vi "GetImage.vi"(0 "XRef":T5, 1 "State In":T3) -> (14 "Image":T2, 15 "Fatal Error Out":T1)   [LabVIEW 2015, in "LVJSON.lvlib" / "Set Object Parameters.xnode"]
uses:
  Set Object Parameters.xnode
  <vilib>/XNodeSupport/XNodeXNodeRef.ctl
  State.ctl
  Get Object Parameters/Parameter.ctl
  <vilib>/XNodeSupport/XNodeImage.ctl
  <vilib>/XNodeSupport/XNodeErrorCluster.ctl
  Shared/Shared.lvlib
  <vilib>/XNodeSupport/NI_XNodeSupport.lvlib
panel:
  in  "picture":picture
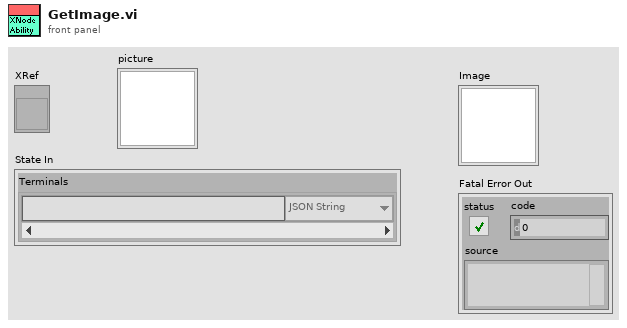
[diagram p1: front panel]
types:
  T1 = typedef "NI_XNodeSupport.lvlib/XNodeErrorCluster.ctl" = errorcluster
  T2 = typedef "NI_XNodeSupport.lvlib/XNodeImage.ctl" = picture
  T3 = typedef "LVJSON.lvlib/Set Object Parameters.xnode/State.ctl" = cluster{"Terminals":T4[]}
  T4 = typedef "LVJSON.lvlib/Shared.lvlib/Parameter.ctl" = cluster{"Parameter Name":string, "JSON Type":enum16{"JSON String", "JSON Numeric", "JSON Boolean", "JSON", "JSON Object", "JSON Array", "String Value", "Numeric Value", "Boolean Value"}}
  T5 = typedef "NI_XNodeSupport.lvlib/XNodeXNodeRef.ctl" = refnum<vi>
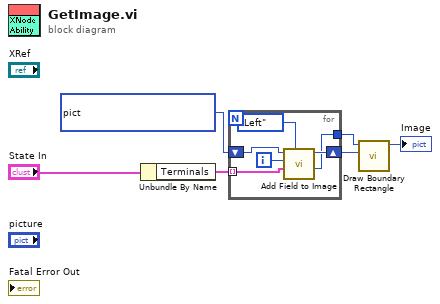
[diagram p0: block diagram]
diagram:
  n1 = Unbundle By Name("State In") -> ("Terminals"=w3:T4[])
  n2 = for {
    shift-right: [w12] -> w5
    shift-left: picture bytes[15070] ("new picture") -> [w11]
    tunnel: w3 -> [w9] mode=indexing
    tunnel: [w8] -> w4
    i -> [w10]
    n3 = call "Add Field to Image.vi"("Justification"=enum16{"Left", "Center", "Right"}."Left", "Terminal Info"=w9, "location"=w10, "picture"=w11) -> ("y"=w8:i16, "new picture"=w12:picture)  [unwired: 6 in]
  }
  n4 = call "Draw Boundary Rectangle.vi"("new picture in"=w5, "y"=w4) -> ("new picture out"=→"Image":picture)  [unwired: 9 in]
